vi "read_converter.vi"(8 "error in (no error)":errorcluster, 11 "VISA Refnum in":refnum<visa-resource-name>) -> (0 "error out":errorcluster, 1 "Types?":cluster{u16, u16, u16, u16, i16}, 2 "sync":bool, 3 "VISA Refnum out":refnum<visa-resource-name>)   [LabVIEW 2019]
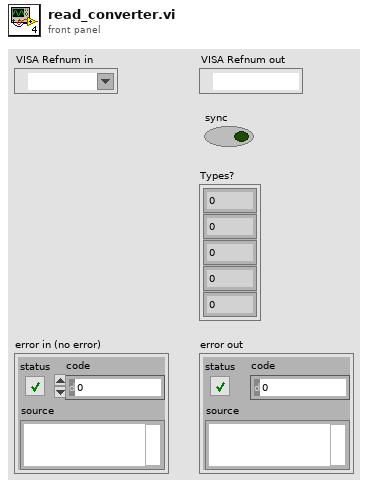
[diagram p1: front panel]
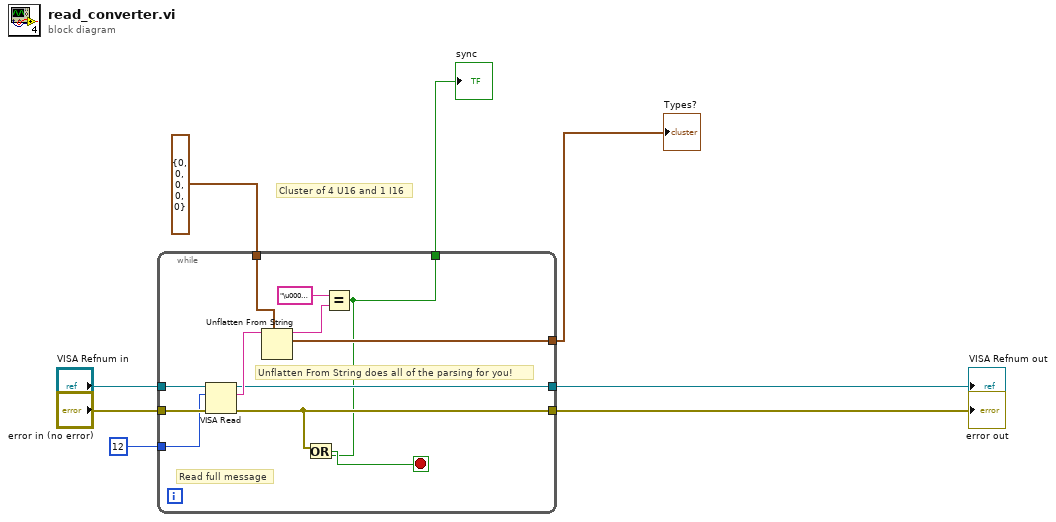
[diagram p0: block diagram]
diagram:
  # "Cluster of 4 U16 and 1 I16"
  n1 = while {
    tunnel: "error in (no error)" -> [w20]
    tunnel: "VISA Refnum in" -> [w19]
    tunnel: [w12] -> w5
    tunnel: [w15] -> w4
    tunnel: [w13] -> w3
    tunnel: cluster{u16, u16, u16, u16, i16} {0, 0, 0, 0, 0} -> [w11]
    tunnel: u32 12 ("byte count") -> [w10]
    tunnel: [w9] -> w8
    stop <- w14 stop-if-true
    # "Unflatten From String does all of the parsing for you!"
    # "Read full message"
    n2 = VISA Read(VISA resource name=w19, byte count=w10, error in (no error)=w20) -> (VISA resource name out=w15:refnum<visa-resource-name>, read buffer=w18:string, error out=w12:errorcluster)  [unwired: 1 out]
    n3 = Unflatten From String(type=w11, binary string=w18) -> (rest of the binary string=w17:string, value=w13:cluster{u16, u16, u16, u16, i16})  [unwired: 3 in, 1 out]
    n4 = Equal?(x="\u0002\u0001", y=w17) -> (x = y?=w9:bool)
    n5 = Or(x=w12, y=w9) -> (x .or. y?=w14:bool)
  }
  "sync" <- w8
  "error out" <- w5
  "VISA Refnum out" <- w4
  "Types?" <- w3
